vi "Round to Nearest.vi"(2 "Input":dbl, 3 "Round to nearest":i32) -> (0 "Output":dbl)   [LabVIEW 2015]
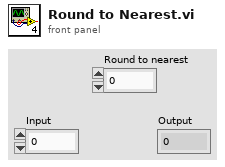
[diagram p1: front panel]
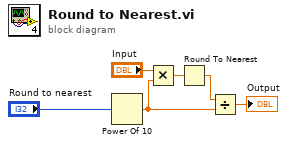
[diagram p0: block diagram]
diagram:
  n1 = Power Of 10(x="Round to nearest") -> (10^x=w3:dbl)
  n2 = Multiply(x="Input", y=w3) -> (x*y=w5:dbl)
  n3 = Round To Nearest(number=w5) -> (nearest integer value=w4:dbl)
  n4 = Divide(x=w4, y=w3) -> (x/y=→"Output":dbl)
